vi "Initialize.vi"(8 "error in":errorcluster, 10 "parameters":variant, 11 "node in":refnum<class "RIO Target.lvclass">) -> (0 "error out":errorcluster, 2 "summary":T2[](array[typedef]), 3 "data value reference":T1)   [LabVIEW 2014, in "RIO Target.lvclass"]
doc: "Initializes the data of a node to its default state.\nThe object is not created inside of this VI, because it is created from a File depending on user selection."
uses:
  RIO Target.lvclass
  <vilib>/NI/Configuration Framework/Node/Summary.ctl
  <vilib>/NI/Configuration Framework/Node/NodeRef.ctl
  <vilib>/NI/Configuration Framework/Node/NISE_CEF_Node.lvclass
  <vilib>/NI/Configuration Framework/serializable node/NISE_CEF_serializable node.lvclass
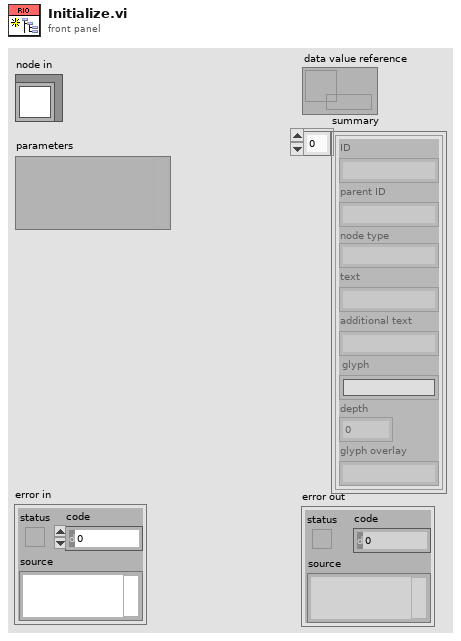
[diagram p1: front panel]
types:
  T1 = typedef "NISE_CEF_Node.lvclass/NodeRef.ctl" = refnum<data-value>
  T2 = typedef "NISE_CEF_Node.lvclass/Summary.ctl" = cluster{"ID":string, "parent ID":string, "node type":string, "text":string, "additional text":string, "glyph":string, "depth":i32, "glyph overlay":string}
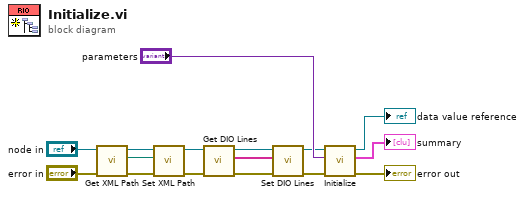
[diagram p0: block diagram]
diagram:
  n1 = call-dynamic "Get XML Path.vi"("error in (no error)"="error in", "RIO Target in"="node in") -> ("error out"=w8:errorcluster, "XML Path"=w10:path, "RIO Target out"=w9:refnum<class "RIO Target.lvclass">)  [unwired: 7 in]
  n2 = call "Set XML Path.vi"("error in (no error)"=w8, "XML Path"=w10, "RIO Target in"=w9) -> ("error out"=w3:errorcluster, "RIO Target out"=w7:refnum<class "RIO Target.lvclass">)  [unwired: 7 in]
  n3 = call "Get DIO Lines.vi"("error in (no error)"=w3, "RIO Target in"=w7) -> ("error out"=w4:errorcluster, "DIO Lines"=w5:string[], "RIO Target out"=w6:refnum<class "RIO Target.lvclass">)  [unwired: 7 in]
  n4 = call "Set DIO Lines.vi"("error in (no error)"=w4, "DIO Lines"=w5, "RIO Target in"=w6) -> ("error out"=w2:errorcluster, "RIO Target out"=w1:refnum<class "RIO Target.lvclass">)  [unwired: 7 in]
  n5 = call-parent "Initialize.vi"("error in"=w2, "parameters"="parameters", "node in"=w1) -> ("error out"=→"error out":errorcluster, "summary"=→"summary":T2[], "data value reference"=→"data value reference":T1)  [unwired: 6 in]
